vi "Replace_data_in_Label_str.vi"(1 "New data string":string, 2 "Input string":string, 3 "Variable name":string) -> (0 "Appended string":string)   [LabVIEW 2010]
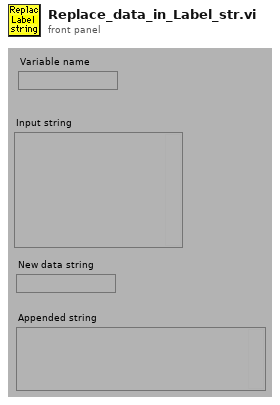
[diagram p1: front panel]
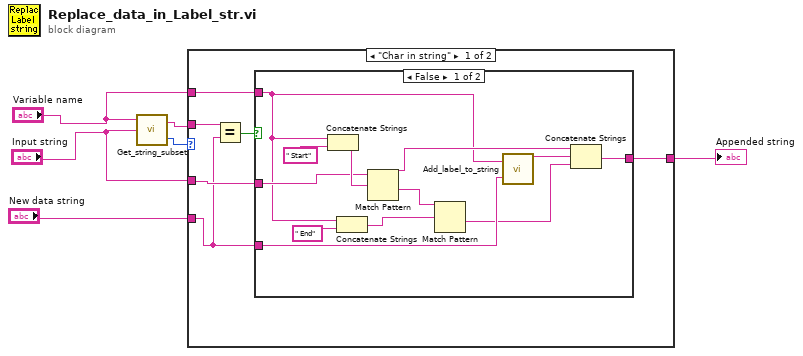
[diagram p0: block diagram]
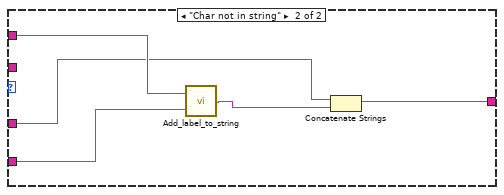
[diagram p3: hidden frame]
diagram:
  n1 = call "Get_string_subset.vi"("String to split"="Input string", "File Label"="Variable name") -> ("Status"=w2:enum16{"Char in string", "Char not in string"}, "Output string"=w1:string)  [unwired: 2 in]
  n2 = case shown="\"Char in string\"" w2 {
    tunnel: "Variable name" -> [w10 w30]
    tunnel: "New data string" -> [w8 w29]
    tunnel: [w11 w28] -> w5
    tunnel: "Input string" -> [w12 w27]
    tunnel: w1 -> [w9 _]
    frame "Char in string" {
      n3 = Equal?(x=w9, y=w8) -> (x = y?=w7:bool)
      n4 = case shown="False" w7 {
        tunnel: w12 -> [w23 w25]
        tunnel: [w22 w25] -> w11
        tunnel: w8 -> [w21 _]
        tunnel: w10 -> [w15 _]
        frame False {
          n5 = Concatenate Strings(w15, " Start") -> (w24:string)
          n6 = Concatenate Strings(w15, " End") -> (w14:string)
          n7 = Match Pattern(string=w23, regular expression=w24) -> (before substring=w19:string, after substring=w17:string)  [unwired: 3 out]
          n8 = Match Pattern(string=w17, regular expression=w14) -> (after substring=w13:string)  [unwired: 4 out]
          n9 = call "Add_label_to_string.vi"("String to write"=w21, "File Label"=w15) -> ("Output string"=w20:string)
          n10 = Concatenate Strings(w19, w20, w13) -> (w22:string)
        }
        frame True {
        }
      }
    }
    frame "Char not in string" {
      n11 = call "Add_label_to_string.vi"("String to write"=w29, "File Label"=w30) -> ("Output string"=w26:string)
      n12 = Concatenate Strings(w27, w26) -> (w28:string)
    }
  }
  "Appended string" <- w5
